vi "Auton Scripting.vi"   [LabVIEW 2014]
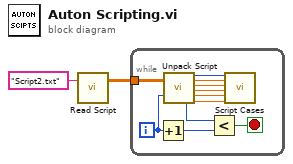
[diagram p0: block diagram]
diagram:
  n1 = call "Read Script.vi"("script name"="Script2.txt") -> ("output array"=w1:dbl[][])  [unwired: 1 in, 1 out]
  n2 = while {
    tunnel: w1 -> [w13]
    i -> [w6]
    stop <- w3 stop-if-true
    n3 = Increment(x=w6) -> (x+1=w4:i32)
    n4 = call "Unpack Script.vi"("script"=w13, "index"=w6) -> ("# of primitives"=w5:i32, "primitive"=w12:i32, "argument 1"=w11:dbl, "argument 2"=w10:dbl, "argument 3"=w9:dbl, "argument 4"=w8:dbl, "argument 5"=w7:dbl)  [unwired: 11 in]
    n5 = Less?(x=w5, y=w4) -> (x < y?=w3:bool)
    n6 = call "Script Cases.vi"("primitive"=w12, "argument 1"=w11, "argument 2"=w10, "argument 3"=w9, "argument 4"=w8, "argument 5"=w7) -> ()  [unwired: 14 in]
  }
